vi "IMAQ-SaveContrast.vi"(1 "contraste":dbl, 2 "tiempo (ms)":u32, 3 "Grabar":refnum<vi>, 4 "Status":string) -> (0 "Archivo de texto":path)   [LabVIEW 2010]
uses:
  <vilib>/Utility/error.llb/DialogType.ctl
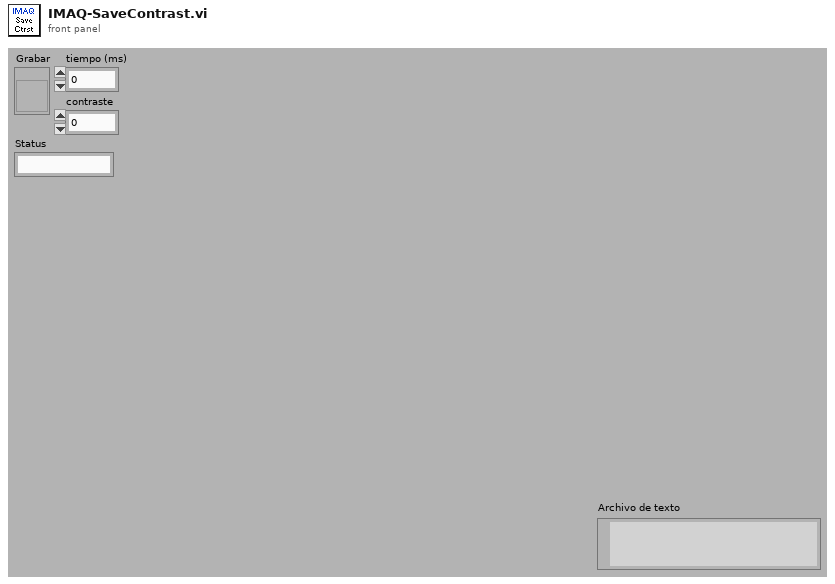
[diagram p1: front panel]
types:
  T1 = enum16{"open", "replace", "create", "open or create", "replace or create", "replace or create with confirmation"}
  T2 = enum32{"existing file", "new file", "new or existing file", "existing dir", "new dir", "new or existing dir", "existing file (use LLBs)", "new file (use LLBs)", "new or existing file (use LLBs)", "new or existing file or directory (use LLBs)"}
  T3 = typedef "DialogType.ctl" = u16
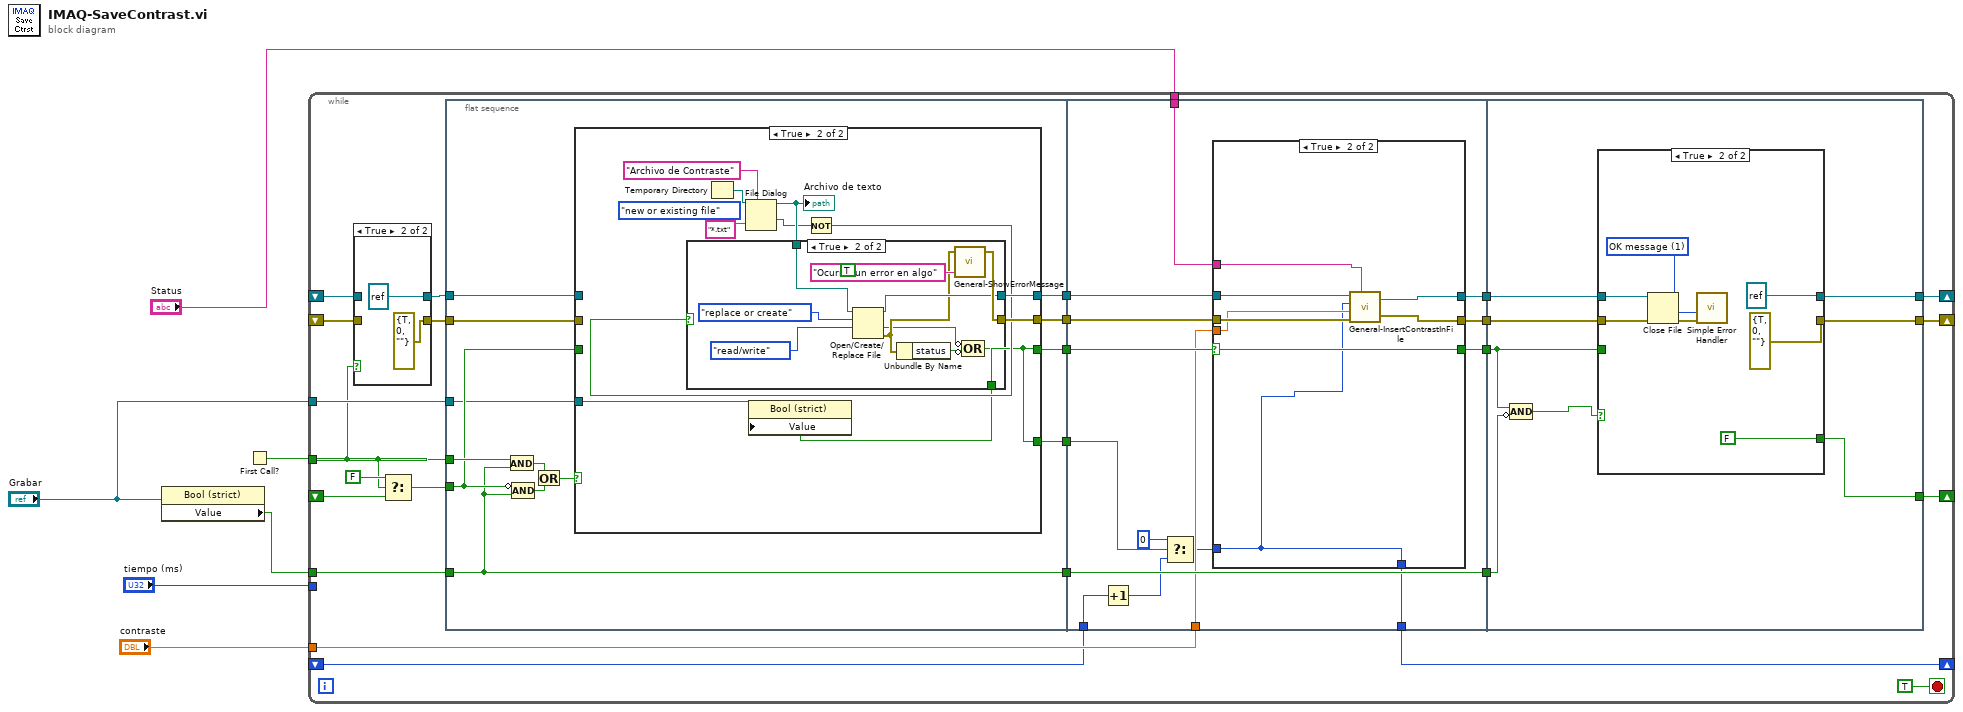
[diagram p0: block diagram]
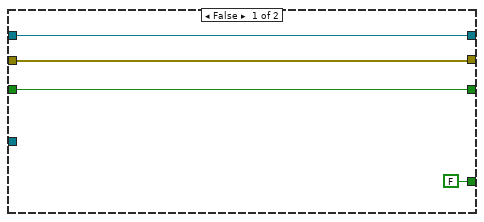
[diagram p3: hidden frame]
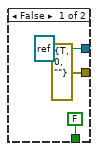
[diagram p4: hidden frame]
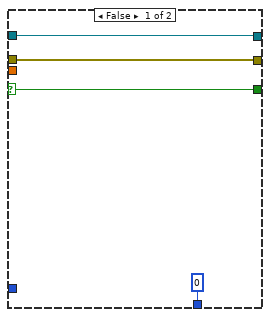
[diagram p5: hidden frame]
diagram:
  n1 = property class="Bool (strict)"(reference="Grabar") -> ("Value"=w5:bool)  [unwired: 1 in, 2 out]
  n2 = First Call?() -> (First Call?: T/F=w6:bool)
  n3 = while {
    tunnel: w6 -> [w8]
    tunnel: w5 -> [w32]
    shift-right: [w18] -> _
    shift-left: _ -> [w30]
    shift-right: [w23] -> _
    shift-left: _ -> [w16]
    shift-right: [w22] -> _
    shift-left: _ -> [w14]
    tunnel: "Grabar" -> [w13]
    tunnel: "tiempo (ms)" -> [_]
    tunnel: "contraste" -> [w12]
    shift-right: [w11] -> _
    shift-left: _ -> [w9]
    tunnel: "Status" -> [w7]
    stop <- TRUE stop-if-true
    n4 = case shown="True" w8 {
      tunnel: [w35 refnum<file> refnum ("refnum OUT")] -> w17
      tunnel: w16 -> [w35 _]
      tunnel: [w34 errorcluster {"status"=TRUE, "code"=0, "source"=""} ("error out")] -> w15
      tunnel: w14 -> [w34 _]
      frame False {
      }
      frame True {
      }
    }
    n5 = Select(t=FALSE, s=w8, f=w30) -> (s? t:f=w29:bool)
    n6 = flat-sequence {
      tunnel: w8 -> [w47]
      tunnel: w32 -> [w40]
      tunnel: w29 -> [w43]
      tunnel: [w46] -> w28
      tunnel: [w45] -> w27
      tunnel: [w44] -> w26
      tunnel: w17 -> [w42]
      tunnel: w15 -> [w41]
      tunnel: [w40] -> w21
      tunnel: w13 -> [w39]
      tunnel: [w38] -> w10
      tunnel: w28 -> [w92]
      tunnel: w27 -> [w85]
      tunnel: w26 -> [w91]
      tunnel: [w90] -> w25
      tunnel: [w89] -> w24
      tunnel: w21 -> [w88]
      tunnel: [w88] -> w20
      tunnel: [w87] -> w19
      tunnel: w12 -> [w86]
      tunnel: [w84] -> w11
      tunnel: w10 -> [w83]
      tunnel: w9 -> [w79]
      tunnel: w7 -> [w78]
      tunnel: w25 -> [w112]
      tunnel: w24 -> [w111]
      tunnel: [w110] -> w23
      tunnel: [w109] -> w22
      tunnel: w20 -> [w108]
      tunnel: w19 -> [w106]
      tunnel: [w107] -> w18
      frame #0 {
        n7 = And(x=w47, y=w40) -> (x .and. y?=w49:bool)
        n8 = Compound Arithmetic op=AND(invert w43, w40) -> (w48:bool)
        n9 = Or(x=w49, y=w48) -> (x .or. y?=w50:bool)
        n10 = case shown="True" w50 {
          tunnel: [w53 w63] -> w46
          tunnel: [w52 w62] -> w45
          tunnel: [w54 w55] -> w44
          tunnel: w43 -> [w54 _]
          tunnel: w42 -> [w52 _]
          tunnel: w41 -> [w53 _]
          tunnel: w39 -> [_ w64]
          tunnel: [FALSE w55] -> w38
          frame False {
          }
          frame True {
            (unwired) T2."new or existing file" ("select mode (2)")
            n11 = Temporary Directory() -> (w59:path)
            n12 = File Dialog(6:"*.txt" ("pattern"), 7:"Archivo de Contraste" ("prompt"), 11:w59) -> (1:w57:bool, 3:w58:path)  [unwired: 1 in, 5 out]
            "Archivo de texto" <- w58
            n13 = Not(x=w57) -> (.not. x?=w56:bool)
            n14 = case shown="True" w56 {
              tunnel: [errorcluster {"status"=TRUE, "code"=0, "source"=""} ("Error OUT") w77] -> w63
              tunnel: w58 -> [_ w75]
              tunnel: [refnum<file> refnum ("refnum out") w72] -> w62
              tunnel: [FALSE w68] -> w55
              frame False {
              }
              frame True {
                (unwired) TRUE ("Has Data")
                n15 = Open/Create/Replace File(file path (use dialog)=w75, operation (0:open)=T1."replace or create", access (0:read/write)=enum16{"read/write", "read-only", "write-only"}."read/write") -> (refnum out=w72:refnum<file>, cancelled=w69:bool, error out=w71:errorcluster)  [unwired: 3 in]
                n16 = Unbundle By Name(w71) -> ("status"=w70:bool)
                n17 = call "General-ShowErrorMessage.vi"("message"="Ocurrio un error en algo", "Error IN"=w71) -> ("Error OUT"=w77:errorcluster)  [unwired: 3 in]
                n18 = Compound Arithmetic op=OR(invert w69, invert w70) -> (w68:bool)
              }
            }
            n19 = property class="Bool (strict)"(reference=w64, "Value"=w55) -> ()  [unwired: 1 in, 2 out]
          }
        }
      }
      frame #1 {
        n20 = Increment(x=w79) -> (x+1=w80:u32)
        n21 = Select(t=u32 0, s=w83, f=w80) -> (s? t:f=w82:u32)
        n22 = case shown="True" w91 {
          selector: w91 -> [w95 w104]
          tunnel: w92 -> [w96 w103]
          tunnel: w85 -> [w94 w99]
          tunnel: [w96 w102] -> w90
          tunnel: [w94 w100] -> w89
          tunnel: [w95 w104] -> w87
          tunnel: w86 -> [_ w101]
          tunnel: w82 -> [_ w98]
          tunnel: [u32 0 ("t") w98] -> w84
          tunnel: w78 -> [_ w97]
          frame False {
          }
          frame True {
            n23 = call "General-InsertContrastInFile.vi"("refnum IN"=w99, "tiempo (ms)"=w98, "contraste"=w101, "error IN"=w103, "Status"=w97) -> ("refnum OUT"=w100:refnum<file>, "error OUT"=w102:errorcluster)
          }
        }
      }
      frame #2 {
        n24 = Compound Arithmetic op=AND(w106, invert w108) -> (w105:bool)
        n25 = case shown="True" w105 {
          tunnel: w112 -> [w114 w121]
          tunnel: w111 -> [w115 w117]
          tunnel: [w115 refnum<file> refnum ("refnum OUT")] -> w110
          tunnel: [w114 errorcluster {"status"=TRUE, "code"=0, "source"=""} ("error out")] -> w109
          tunnel: [w113 FALSE] -> w107
          tunnel: w106 -> [w113 _]
          frame False {
          }
          frame True {
            w118 = T3 1 items=["no dialog", "OK message", "continue or stop message", "OK message + warnings", "continue/stop + warnings"] ("type of dialog (OK msg:1)")
            n26 = Close File(refnum=w117, error in=w121) -> (error out=w122:errorcluster)  [unwired: 1 out]
            n27 = call <vilib>:"Simple Error Handler.vi"("type of dialog (OK msg:1)"=w118, "error in (no error)"=w122) -> ()  [unwired: 8 out]
          }
        }
      }
    }
  }
